vi "Test Calibrate.vi"() -> ()   [LabVIEW 2012]
uses:
  <vilib>/Instr/_visa.llb/VISA Flush IO Buffer Mask.ctl
  <vilib>/Platform/TimedLoop/XDataNode/timing_clust.ctl
  <vilib>/Platform/TimedLoop/XDataNode/nitl_modes.ctl
  <vilib>/Platform/TimedLoop/XDataNode/wakeup.ctl
  <vilib>/platform/TimedLoop/XDataNode/XDataNode.xnode
  <vilib>/Platform/TimedLoop/XDataNode/XDNodeRunTimeDep.lvlib
panel:
  out "read buffer":string
  out "error out":errorcluster
  out "Version":string
  out "trimmed string":string
  in  "Stop":bool
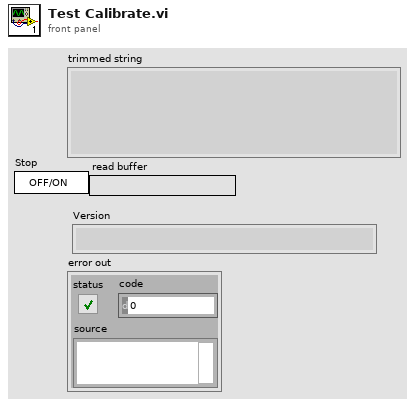
[diagram p1: front panel]
types:
  T1 = typedef "XDNodeRunTimeDep.lvlib/timing_clust.ctl" = cluster{"Expected End [f-1]":u64, "Actual End [f-1]":u64, "Finished Late? [f-1]":bool, "Expected End [i-1]":u64, "Actual End [i-1]":u64, "Finished Late? [i-1]":bool, "Expected Start [i]":u64, "Actual Start [i]":u64, "Expected Start [f]":u64, "Actual Start [f]":u64, "Source Name":string, "Structure Name":string, "Period":i64, "Deadline":i64, "Offset":i64, "Start":i64, "Priority":i32, "Timeout":i32, "Mode":T2, "Wakeup Reason":T3, "Error":errorcluster, "Source Type":string, "Secondary Source Type":string, "Global End Time":u64, "Global Start Time":u64, "Frame Duration":u64, "Iteration Duration":u64, "Assigned CPU":i32, "I/O Scan Engine Mode":u32}
  T2 = typedef "XDNodeRunTimeDep.lvlib/nitl_modes.ctl" = enum32{"No Change", "Process missed periods, maintain original phase", "Discard missed periods, maintain original phase", "Process missed periods, ignore original phase", "Discard missed periods, ignore original phase"}
  T3 = typedef "XDNodeRunTimeDep.lvlib/wakeup.ctl" = enum32{"Normal", "Aborted", "Asynchronous wakeup", "Timing source error", "Timed loop error", "Timeout"}
  T4 = typedef "VISA Flush IO Buffer Mask.ctl" = u16
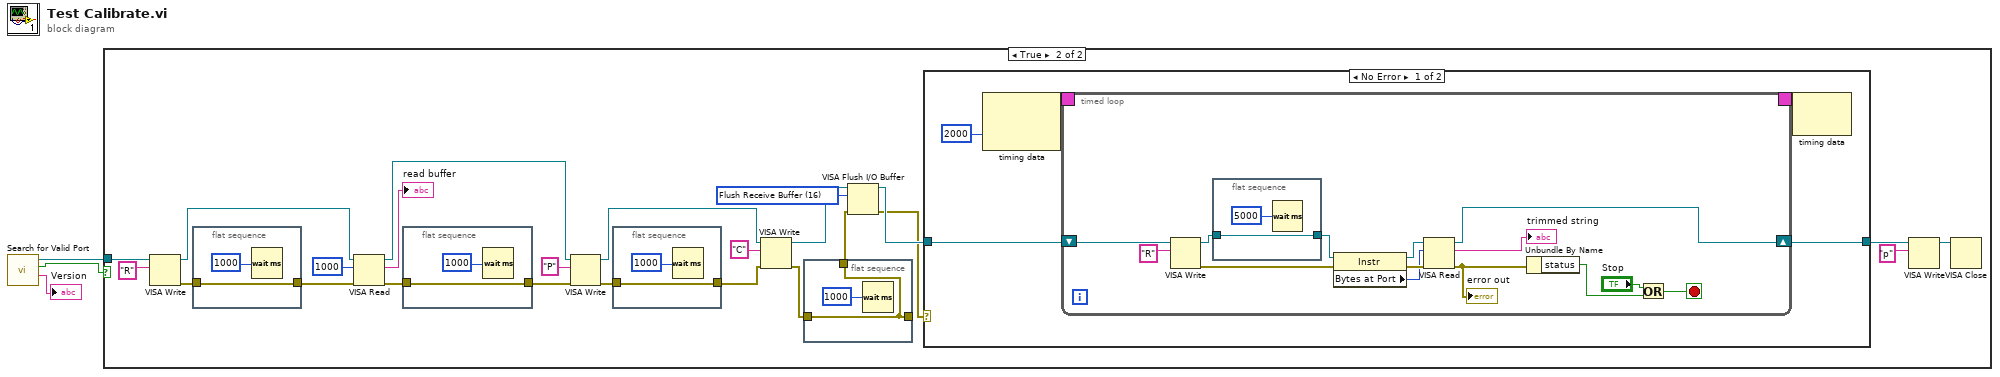
[diagram p0: block diagram]
diagram:
  n1 = call "Search for Valid Port.vi"() -> ("Version"=→"Version":string, "CAT Port?"=w3:bool, "Port Out"=w2:refnum<visa-resource-name>)  [unwired: 9 in]
  n2 = case shown="True" w3 {
    tunnel: w2 -> [_ w10]
    frame False {
    }
    frame True {
      w7 = T4 16 items=["Flush Receive Buffer"=16, "Write Transmit Buffer to Device"=32, "Flush Receive Buffer (No I/O)"=64, "Flush Transmit Buffer"=128] ("Mask")
      n3 = VISA Write(VISA resource name=w10, write buffer="R") -> (VISA resource name out=w17:refnum<visa-resource-name>, error out=w16:errorcluster)  [unwired: 1 in, 1 out]
      n4 = flat-sequence {
        tunnel: w16 -> [w28]
        tunnel: [w28] -> w15
        frame #0 {
          n5 = Wait (ms)(milliseconds to wait=u32 1000) -> ()  [unwired: 1 out]
        }
      }
      n6 = VISA Read(VISA resource name=w17, byte count=u32 1000, error in (no error)=w15) -> (VISA resource name out=w9:refnum<visa-resource-name>, read buffer=→"read buffer":string, error out=w14:errorcluster)  [unwired: 1 out]
      n7 = flat-sequence {
        tunnel: w14 -> [w30]
        tunnel: [w30] -> w13
        frame #0 {
          n8 = Wait (ms)(milliseconds to wait=u32 1000) -> ()  [unwired: 1 out]
        }
      }
      n9 = VISA Write(VISA resource name=w9, write buffer="P", error in (no error)=w13) -> (VISA resource name out=w11:refnum<visa-resource-name>, error out=w21:errorcluster)  [unwired: 1 out]
      n10 = flat-sequence {
        tunnel: w21 -> [w34]
        tunnel: [w34] -> w12
        frame #0 {
          n11 = Wait (ms)(milliseconds to wait=u32 1000) -> ()  [unwired: 1 out]
        }
      }
      n12 = VISA Write(VISA resource name=w11, write buffer="C", error in (no error)=w12) -> (VISA resource name out=w8:refnum<visa-resource-name>, error out=w26:errorcluster)  [unwired: 1 out]
      n13 = flat-sequence {
        tunnel: w26 -> [w32]
        tunnel: [w32] -> _
        tunnel: [w32] -> w5
        frame #0 {
          n14 = Wait (ms)(milliseconds to wait=u32 1000) -> ()  [unwired: 1 out]
        }
      }
      n15 = VISA Flush I/O Buffer(VISA resource name=w8, mask (16)=w7, error in (no error)=w5) -> (VISA resource name out=w6:refnum<visa-resource-name>, error out=w4:errorcluster)
      n16 = case shown="No Error" w4 {
        tunnel: [w38 w63] -> w24
        tunnel: w6 -> [w36 w63]
        frame No Error {
          n17 = node-c288(i64 2000 ("Period")) -> (w40:T1)  [unwired: 1 in]
          n18 = timed-loop {
            timing: w40 -> [_]
            timing-out: [_] -> w39
            shift-right: [w42] -> w38
            shift-left: w36 -> [w41]
            stop <- w43 stop-if-true
            n19 = VISA Write(VISA resource name=w41, write buffer="R") -> (VISA resource name out=w53:refnum<visa-resource-name>, error out=w51:errorcluster)  [unwired: 1 in, 1 out]
            n20 = flat-sequence {
              tunnel: w53 -> [w55]
              tunnel: [w55] -> w52
              frame #0 {
                n21 = Wait (ms)(milliseconds to wait=u32 5000) -> ()  [unwired: 1 out]
              }
            }
            n22 = property class="Instr"(reference=w52, error in=w51) -> (reference out=w50:refnum<visa-resource-name>, error out=w49:errorcluster, "Bytes at Port"=w48:u32)
            n23 = VISA Read(VISA resource name=w50, byte count=w48, error in (no error)=w49) -> (VISA resource name out=w42:refnum<visa-resource-name>, read buffer=→"trimmed string":string, error out=w45:errorcluster)  [unwired: 1 out]
            "error out" <- w45
            n24 = Unbundle By Name(w45) -> ("status"=w44:bool)
            n25 = Or(x="Stop", y=w44) -> (x .or. y?=w43:bool)
          }
          n26 = node-c288(w39) -> ()  [unwired: 1 out]
        }
        frame Error {
        }
      }
      n27 = VISA Write(VISA resource name=w24, write buffer="p") -> (VISA resource name out=w23:refnum<visa-resource-name>)  [unwired: 1 in, 2 out]
      n28 = VISA Close(VISA resource name=w23) -> ()  [unwired: 1 in, 1 out]
    }
  }
